vi "relative access path.vi"(11 "Oauth2.Github":refnum<class "Oauth2.GitHub.lvclass">) -> (1 "Token Access Path":string, 2 "Authorization Path":string)   [LabVIEW 2020, in "Oauth2.GitHub.lvclass"]
uses:
  Oauth2.GitHub.lvclass
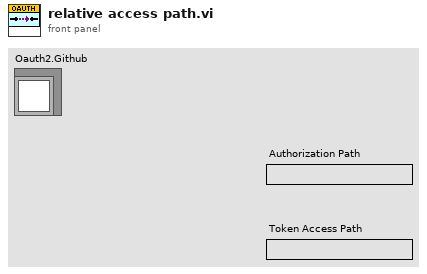
[diagram p1: front panel]
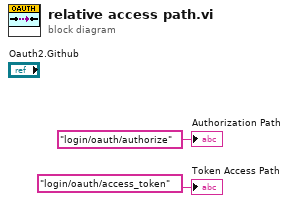
[diagram p0: block diagram]
diagram:
  "Authorization Path" <- "login/oauth/authorize" ("Authorization Path")
  "Token Access Path" <- "login/oauth/access_token" ("Authorization Path")
